vi "_RT_CtrlLoop_Pressure_Read_VISA.vi"(8 "error in (no error)":errorcluster, 10 "Comm Str":string, 11 "VISA resource In":refnum<visa-resource-name>) -> (0 "error out":errorcluster, 2 "Response Str":string, 3 "VISA resource Out":refnum<visa-resource-name>)   [LabVIEW 2018]
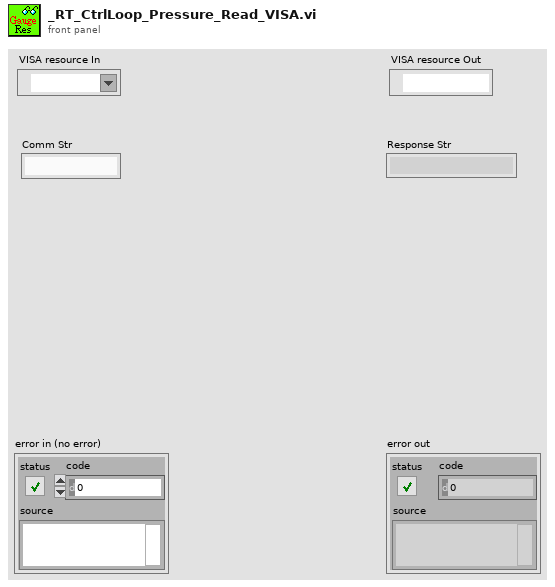
[diagram p1: front panel]
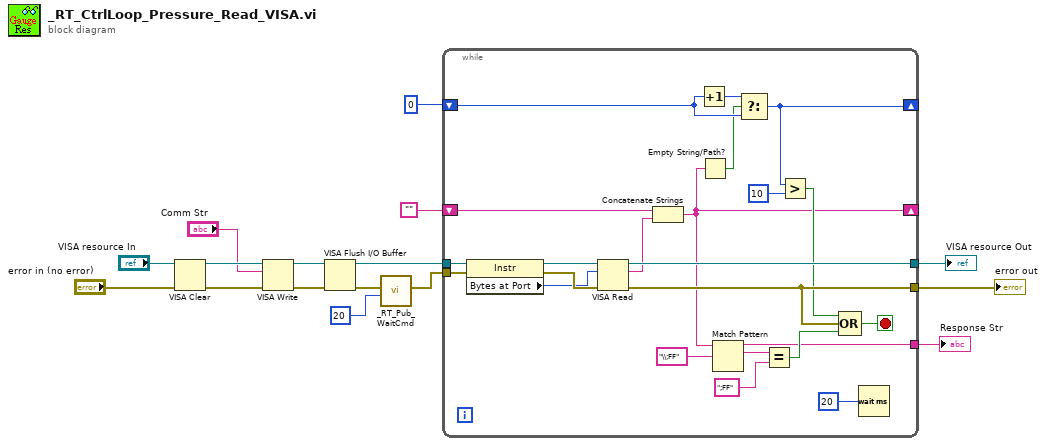
[diagram p0: block diagram]
diagram:
  n1 = VISA Clear(VISA resource name="VISA resource In", error in (no error)="error in (no error)") -> (VISA resource name out=w11:refnum<visa-resource-name>, error out=w10:errorcluster)
  n2 = VISA Write(VISA resource name=w11, write buffer="Comm Str", error in (no error)=w10) -> (VISA resource name out=w5:refnum<visa-resource-name>, error out=w4:errorcluster)  [unwired: 1 out]
  n3 = VISA Flush I/O Buffer(VISA resource name=w5, error in (no error)=w4) -> (VISA resource name out=w3:refnum<visa-resource-name>, error out=w2:errorcluster)  [unwired: 1 in]
  n4 = call "_RT_Pub_WaitCmd.vi"("milliseconds to wait"=u32 20, "error in (no error)"=w2) -> ("error out"=w8:errorcluster)  [unwired: 9 in]
  n5 = while {
    shift-right: [w17] -> _
    shift-left: "" -> [w20]
    tunnel: [w39] -> w14
    tunnel: [w35] -> w13
    tunnel: w3 -> [w30]
    tunnel: w8 -> [w29]
    tunnel: [w25] -> w6
    shift-right: [w21] -> _
    shift-left: 0 -> [w22]
    stop <- w33 stop-if-true
    n6 = property class="Instr"(reference=w30, error in=w29) -> (reference out=w31:refnum<visa-resource-name>, error out=w32:errorcluster, "Bytes at Port"=w28:u32)
    n7 = VISA Read(VISA resource name=w31, byte count=w28, error in (no error)=w32) -> (VISA resource name out=w39:refnum<visa-resource-name>, read buffer=w26:string, error out=w35:errorcluster)  [unwired: 1 out]
    n8 = Concatenate Strings(w20, w26) -> (w17:string)
    n9 = Increment(x=w22) -> (x+1=w24:i32)
    n10 = Empty String/Path?(string/path=w17) -> (empty?=w19:bool)
    n11 = Match Pattern(string=w17, regular expression="\\;FF") -> (before substring=w25:string, match substring=w37:string)  [unwired: 1 in, 2 out]
    n12 = Select(t=w24, s=w19, f=w22) -> (s? t:f=w21:i32)
    n13 = Equal?(x=w37, y=";FF") -> (x = y?=w34:bool)
    n14 = Greater?(x=w21, y=10) -> (0:w18:bool)
    n15 = Compound Arithmetic op=OR(w18, w35, w34) -> (w33:bool)
    n16 = Wait (ms)(milliseconds to wait=u32 20) -> ()  [unwired: 1 out]
  }
  "error out" <- w13
  "VISA resource Out" <- w14
  "Response Str" <- w6
